vi "Query PRT Data.vi"(8 "error in (no error)":errorcluster, 11 "VISA resource name":refnum<visa-resource-name>) -> (0 "error out":errorcluster, 2 "PRT Probe Data":T1(array[cluster]), 3 "VISA resource name out":refnum<visa-resource-name>)   [LabVIEW 2011, in "Fluke 8508.lvlib"]
doc: "This VI queries and displays the characteristics of all the PRT probes stored on the instrument."
uses:
  Fluke 8508.lvlib
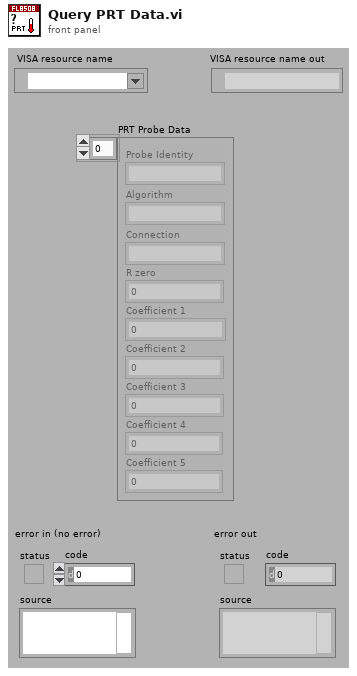
[diagram p1: front panel]
types:
  T1 = cluster{"Probe Identity":string, "Algorithm":string, "Connection":string, "R zero":dbl, "Coefficient 1":dbl, "Coefficient 2":dbl, "Coefficient 3":dbl, "Coefficient 4":dbl, "Coefficient 5":dbl}[]
  T2 = cluster{"Probe Identity":string, "Algorithm":string, "Connection":string, "R zero":dbl, "Coefficient 1":dbl, "Coefficient 2":dbl, "Coefficient 3":dbl, "Coefficient 4":dbl, "Coefficient 5":dbl}
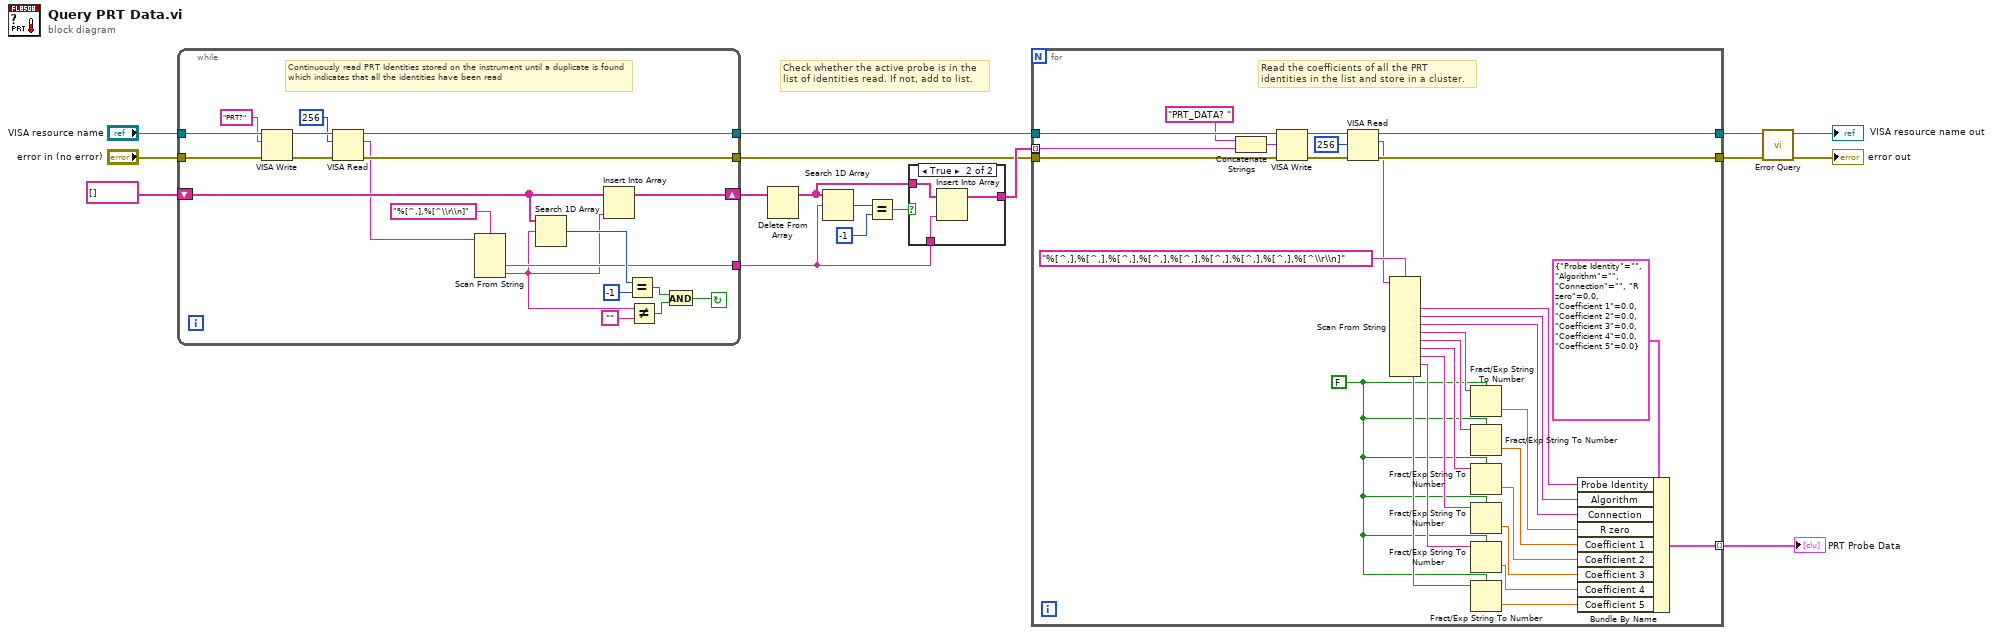
[diagram p0: block diagram]
diagram:
  # "Check whether the active probe is in the list of identities read. If not, add to list."
  n1 = while {
    tunnel: "VISA resource name" -> [w37]
    tunnel: "error in (no error)" -> [w36]
    tunnel: [w31] -> w5
    tunnel: [w30] -> w4
    shift-right: [w24] -> w12
    shift-left: string[] [] -> [w26]
    tunnel: [w25] -> w7
    stop <- w20 continue-if-true
    # "Continuously read PRT Identities stored on the instrument until a duplicate is found which indicates that all the identities have been read"
    n2 = VISA Write(VISA resource name=w37, write buffer="PRT?", error in (no error)=w36) -> (VISA resource name out=w35:refnum<visa-resource-name>, error out=w34:errorcluster)  [unwired: 1 out]
    n3 = VISA Read(VISA resource name=w35, byte count=u32 256, error in (no error)=w34) -> (VISA resource name out=w31:refnum<visa-resource-name>, read buffer=w23:string, error out=w30:errorcluster)  [unwired: 1 out]
    n4 = Scan From String(format string="%[^,],%[^\\r\\n]", input string=w23) -> (output 1=w25:string, output 2=w19:string)  [unwired: 4 in, 3 out]
    n5 = Search 1D Array(1D array=w26, element=w19) -> (index of element=w28:i32)  [unwired: 1 in]
    n6 = Insert Into Array(array=w26, new element=w19) -> (w24:string[])  [unwired: 1 in]
    n7 = Equal?(x=w28, y=-1) -> (x = y?=w21:bool)
    n8 = Not Equal?(x=w19, y="") -> (x != y?=w22:bool)
    n9 = And(x=w21, y=w22) -> (x .and. y?=w20:bool)
  }
  n10 = Delete From Array(array=w12) -> (array with subset deleted=w9:string[])  [unwired: 2 in, 1 out]
  n11 = Search 1D Array(1D array=w9, element=w7) -> (index of element=w11:i32)  [unwired: 1 in]
  n12 = Equal?(x=w11, y=-1) -> (x = y?=w8:bool)
  n13 = case shown="True" w8 {
    tunnel: w9 -> [w38 w41]
    tunnel: w7 -> [_ w40]
    tunnel: [w38 w39] -> w6
    frame False {
    }
    frame True {
      n14 = Insert Into Array(array=w41, new element=w40) -> (w39:string[])  [unwired: 1 in]
    }
  }
  n15 = for {
    tunnel: w6 -> [w57] mode=indexing
    tunnel: w5 -> [w70]
    tunnel: w4 -> [w69]
    tunnel: [w66] -> w3
    tunnel: [w65] -> w2
    tunnel: [w56] -> w1 mode=indexing
    w48 = FALSE ("use system decimal point (T)")
    # "Read the coefficients of all the PRT identities in the list and store in a cluster."
    n16 = Concatenate Strings("PRT_DATA? ", w57) -> (w64:string)
    n17 = VISA Write(VISA resource name=w70, write buffer=w64, error in (no error)=w69) -> (VISA resource name out=w68:refnum<visa-resource-name>, error out=w71:errorcluster)  [unwired: 1 out]
    n18 = VISA Read(VISA resource name=w68, byte count=u32 256, error in (no error)=w71) -> (VISA resource name out=w66:refnum<visa-resource-name>, read buffer=w55:string, error out=w65:errorcluster)  [unwired: 1 out]
    n19 = Scan From String(format string="%[^,],%[^,],%[^,],%[^,],%[^,],%[^,],%[^,],%[^,],%[^\\r\\n]", input string=w55) -> (output 1=w60:string, output 2=w59:string, output 3=w58:string, output 4=w54:string, output 5=w53:string, output 6=w52:string, output 7=w51:string, output 8=w50:string, output 9=w49:string)  [unwired: 11 in, 3 out]
    n20 = Fract/Exp String To Number(use system decimal point (T)=w48, string=w54) -> (number=w42:dbl)  [unwired: 2 in, 1 out]
    n21 = Fract/Exp String To Number(use system decimal point (T)=w48, string=w53) -> (number=w43:dbl)  [unwired: 2 in, 1 out]
    n22 = Fract/Exp String To Number(use system decimal point (T)=w48, string=w52) -> (number=w44:dbl)  [unwired: 2 in, 1 out]
    n23 = Fract/Exp String To Number(use system decimal point (T)=w48, string=w51) -> (number=w45:dbl)  [unwired: 2 in, 1 out]
    n24 = Fract/Exp String To Number(use system decimal point (T)=w48, string=w50) -> (number=w46:dbl)  [unwired: 2 in, 1 out]
    n25 = Fract/Exp String To Number(use system decimal point (T)=w48, string=w49) -> (number=w47:dbl)  [unwired: 2 in, 1 out]
    n26 = Bundle By Name(cluster=T2 {"Probe Identity"="", "Algorithm"="", "Connection"="", "R zero"=0.0, "Coefficient 1"=0.0, "Coefficient 2"=0.0, "Coefficient 3"=0.0, "Coefficient 4"=0.0, "Coefficient 5"=0.0} ("input cluster"), "Probe Identity"=w60, "Algorithm"=w59, "Connection"=w58, "R zero"=w42, "Coefficient 1"=w43, "Coefficient 2"=w44, "Coefficient 3"=w45, "Coefficient 4"=w46, "Coefficient 5"=w47) -> (w56:T2)
  }
  "PRT Probe Data" <- w1
  n27 = call "Error Query.vi"("error in (no error)"=w2, "VISA resource name"=w3) -> ("error out"=→"error out":errorcluster, "VISA resource name out"=→"VISA resource name out":refnum<visa-resource-name>)  [unwired: 6 in, 2 out]
